vi "table content size.vi"(7 "border (0px)":i32, 8 "error in (no error)":errorcluster, 9 "#columns":i32, 10 "#rows":i32, 11 "table":refnum<vi>) -> (0 "error out":errorcluster, 2 "Size":T1, 3 "table":refnum<vi>)   [LabVIEW 2021, in "RocketPlot.lvlib" / "TipTablePanel.lvclass"]
uses:
  TipTablePanel.lvclass
  <vilib>/Utility/miscctls.llb/LVBoundsTypeDef.ctl
  <vilib>/Utility/miscctls.llb/LVRowAndColumnTypeDef.ctl
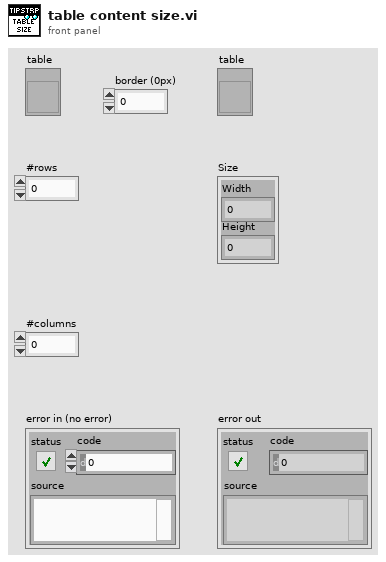
[diagram p1: front panel]
types:
  T1 = typedef "LVBoundsTypeDef.ctl" = cluster{"Width":u32, "Height":u32}
  T2 = typedef "LVRowAndColumnTypeDef.ctl" = cluster{"Row":i32, "Column":i32}
  T3 = typedef "LVPositionTypeDef.ctl" = cluster{"Left":i32, "Top":i32}
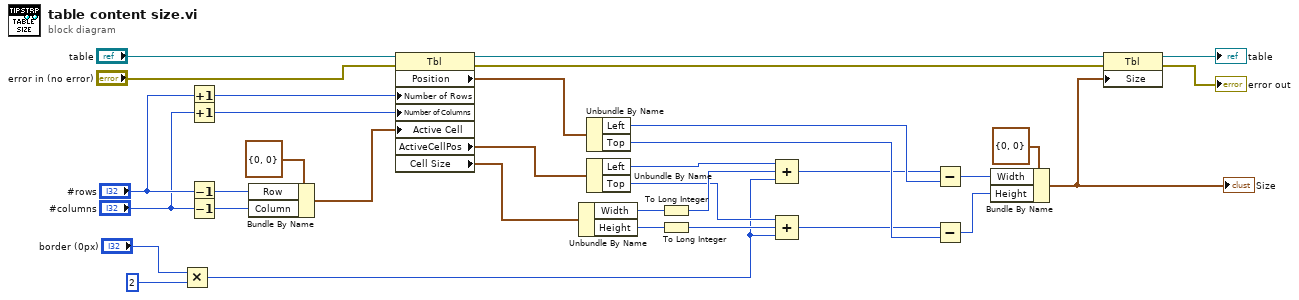
[diagram p0: block diagram]
diagram:
  n1 = Multiply(x="border (0px)", y=2) -> (x*y=w1:i32)
  n2 = Increment(x="#rows") -> (x+1=w12:i32)
  n3 = Increment(x="#columns") -> (x+1=w10:i32)
  n4 = Decrement(x="#rows") -> (x-1=w24:i32)
  n5 = Decrement(x="#columns") -> (x-1=w23:i32)
  n6 = Bundle By Name(cluster=T2 {"Row"=0, "Column"=0} ("Active Cell:Active Cell"), "Row"=w24, "Column"=w23) -> (w15:T2)
  n7 = property class="Tbl"(reference="table", error in="error in (no error)", "Number of Rows"=w12, "Number of Columns"=w10, "Active Cell"=w15) -> (reference out=w14:refnum<vi>, error out=w22:errorcluster, "Position"=w28:T3, "ActiveCellPos"=w32:T3, "Cell Size"=w31:T1)
  n8 = Unbundle By Name(w31) -> ("Width"=w30:u32, "Height"=w29:u32)
  n9 = Unbundle By Name(w28) -> ("Left"=w27:i32, "Top"=w26:i32)
  n10 = Unbundle By Name(w32) -> ("Left"=w7:i32, "Top"=w4:i32)
  n11 = To Long Integer(number=w30) -> (32bit integer=w6:i32)
  n12 = To Long Integer(number=w29) -> (32bit integer=w3:i32)
  n13 = Compound Arithmetic op=ADD(w7, w6, w1) -> (w5:i32)
  n14 = Compound Arithmetic op=ADD(w4, w3, w1) -> (w2:i32)
  n15 = Subtract(x=w5, y=w27) -> (x-y=w19:i32)
  n16 = Subtract(x=w2, y=w26) -> (x-y=w18:i32)
  n17 = Bundle By Name(cluster=T1 {"Width"=0, "Height"=0} ("Size"), "Width"=w19, "Height"=w18) -> (w16:T1)
  "Size" <- w16
  n18 = property class="Tbl"(reference=w14, error in=w22, "Size"=w16) -> (reference out=→"table":refnum<vi>, error out=→"error out":errorcluster)
